vi "Function_reset.vi"(5 "VISA resource name in":refnum<visa-resource-name>, 7 "error in":errorcluster, 11 "Server addr":string) -> (4 "VISA resource name out":refnum<visa-resource-name>, 6 "error out":errorcluster)   [LabVIEW 2020]
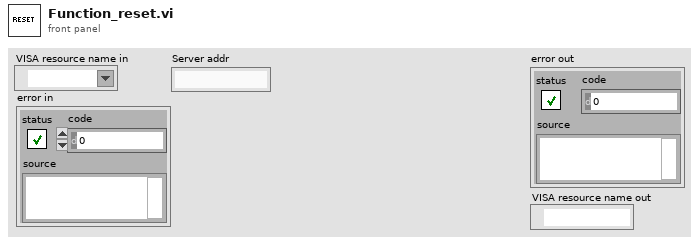
[diagram p1: front panel]
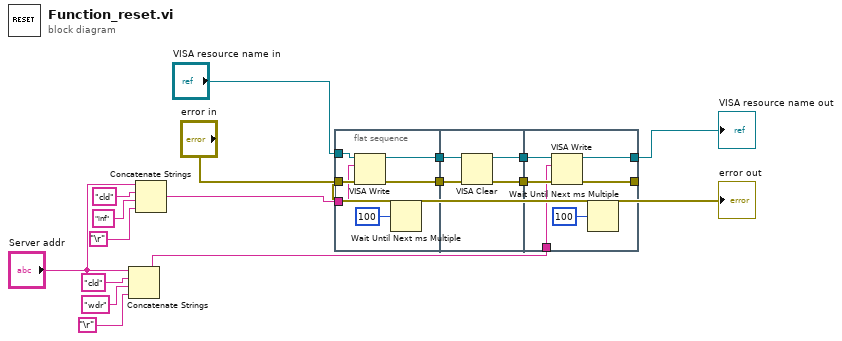
[diagram p0: block diagram]
diagram:
  n1 = Concatenate Strings("Server addr", "cld" ("string"), "wdr" ("string"), "\r") -> (w6:string)
  n2 = Concatenate Strings("Server addr", "cld" ("string"), "inf" ("string"), "\r") -> (w12:string)
  n3 = flat-sequence {
    tunnel: w12 -> [w23]
    tunnel: "VISA resource name in" -> [w22]
    tunnel: "error in" -> [w21]
    tunnel: [w20] -> w17
    tunnel: [w19] -> w16
    tunnel: w17 -> [w26]
    tunnel: w16 -> [w27]
    tunnel: [w25] -> w15
    tunnel: [w24] -> w14
    tunnel: [w30] -> w1
    tunnel: [w31] -> w2
    tunnel: w15 -> [w32]
    tunnel: w14 -> [w33]
    tunnel: w6 -> [w28]
    frame #0 {
      n4 = VISA Write(VISA resource name=w22, write buffer=w23, error in (no error)=w21) -> (VISA resource name out=w20:refnum<visa-resource-name>, error out=w19:errorcluster)  [unwired: 1 out]
      n5 = Wait Until Next ms Multiple(millisecond multiple=u32 100) -> ()  [unwired: 1 out]
    }
    frame #1 {
      n6 = VISA Clear(VISA resource name=w26, error in (no error)=w27) -> (VISA resource name out=w25:refnum<visa-resource-name>, error out=w24:errorcluster)
    }
    frame #2 {
      n7 = VISA Write(VISA resource name=w32, write buffer=w28, error in (no error)=w33) -> (VISA resource name out=w31:refnum<visa-resource-name>, error out=w30:errorcluster)  [unwired: 1 out]
      n8 = Wait Until Next ms Multiple(millisecond multiple=u32 100) -> ()  [unwired: 1 out]
    }
  }
  "error out" <- w1
  "VISA resource name out" <- w2
